vi "Process.vi"(8 "error in":errorcluster, 11 "Instrument.Cryostation UI":refnum<class "Instrument UI.Cryostation.lvclass">) -> (0 "error out":errorcluster, 3 "Instrument.Cryostation UI":refnum<class "Instrument UI.Cryostation.lvclass">)   [LabVIEW 2020, in "Instrument UI.Cryostation.lvclass"]
doc: "---------------------------------------------------------------\nJKI State Machine Objects™\nhttp://jki.net/state-machine-objects/\nCopyright (C) 2005-2015, JKI <info@jki.net>\nALL RIGHTS RESERVEDJKI State Machine Objects (SMO) 1.0.0.5\nJKI - JKI\nCopyright (c) 2016, JKI"
uses:
  Instrument UI.Cryostation.lvclass
  C:/Program Files (x86)/National Instruments/LabVIEW 2020/vi.lib/JKI/JKI SMO/SMO/SMO.lvclass
  C:/Program Files (x86)/National Instruments/LabVIEW 2020/user.lib/LevyLab/Instrument Framework/Instrument UI/Instrument UI.lvclass
  C:/Program Files (x86)/National Instruments/LabVIEW 2020/vi.lib/JKI/JKI SMO/SMO.UI/SMO.UI.lvclass
  instrument.Cryostation/Typedefs/Cryostation.getAll--cluster.ctl
  instrument.Cryostation/instrument.Cryostation.lvclass
  C:/Program Files (x86)/National Instruments/LabVIEW 2020/user.lib/LevyLab/Instrument Framework/Instrument/Instrument.lvclass
  <userlib>/LevyLab/Instrument Framework/Instrument UI/Instrument UI.lvclass/Instrument UI.ctl
  instrument.Cryostation/instrument.Cryostation.lvclass/instrument.Cryostation.ctl
  <vilib>/JKI/JKI SMO/SMO/SMO.lvclass/SMO.ctl
  fdd1bc94-5494-416e-8b24-9b7f0f20f078.vi
  fdd1bc94-5494-416e-8b24-9b7f0f20f078.vi/9c58c222-23e3-43d9-b644-b9682e939e3b.vi
  fdd1bc94-5494-416e-8b24-9b7f0f20f078.vi/ae596761-01aa-4433-afa8-424f3b97f88e.vi
  <vilib>/JKI/JKI SMO/SMO/Private/ReftoDVR--SMO.vi
  <vilib>/Utility/Data Type/Get Type Information.vi
  <vilib>/JDP Science/JSONtext/JSON text to Variant.vi
  <vilib>/JDP Science/JSONtext/LVClass Serializer/JSONtext LVClass Serializer.lvclass
  <userlib>/LevyLab/Instrument Framework/Instrument/Instrument.lvclass
  <userlib>/LevyLab/Instrument Framework/Instrument UI/Instrument UI.lvclass
  Instrument UI.Cryostation.lvclass/Instrument UI.Cryostation.ctl
  <vilib>/JKI/JKI SMO/SMO/SMO.lvclass
  <vilib>/JKI/JKI SMO/SMO.UI/SMO.UI.lvclass
  <userlib>/_OpenG.lib/appcontrol/appcontrol.llb/openg_application_control.lvlib
  D:/Montana-Instruments-Cryostation/lvsrc/instrument.Cryostation UI/Instrument UI.Cryostation.lvclass
  C:/Program Files (x86)/National Instruments/LabVIEW 2020/user.lib/LevyLab/Instrument Framework/Instrument Types/Cryostat/Instrument.Cryostat.lvclass
  D:/Montana-Instruments-Cryostation/lvsrc/instrument.Cryostation/instrument.Cryostation.lvclass
panel:
  out "version":string
  out "Chamber Pressure (mTorr)":dbl=305.0156 format="%#_5f"
  out "Stage 2 Temperature (K)":dbl=305.0156 format="%#_5f"
  out "Stage 1 Temperature (K)":dbl=305.0156 format="%#_5f"
  out "Sample Temperature (K)":dbl=305.0156 format="%#_5f"
  out "Platform Temperature (K)":dbl=305.0156 format="%#_5f"
  # "Cryostation Monitor and Control"
  # "SMO UI Template"
  # "For instructions on how to use the JKI State Machine Objects, examples and video tutorials, visit:\nhttp://jki.net/state-machine-objects/\n\nJKI State Machine Objects™\nhttp://jki.net/state-machine-objects/\nCopyright (C) 2005-2015, JKI <info@jki.net>\nALL RIGHTS RESERVED"
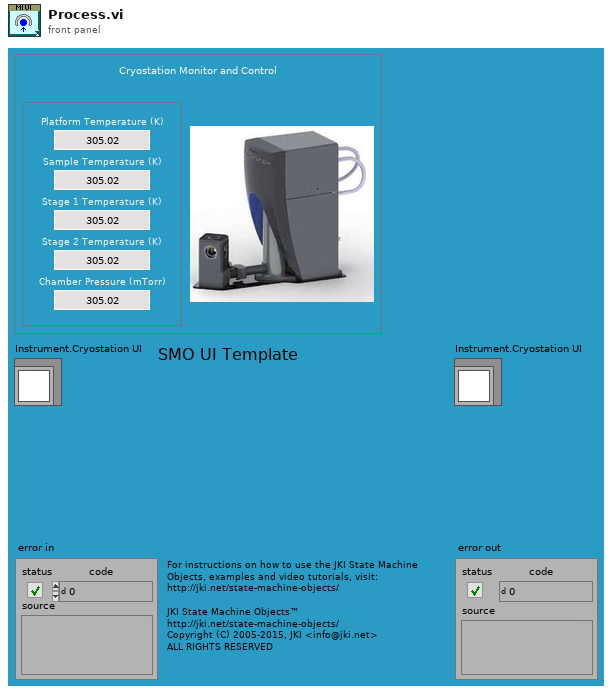
[diagram p1: front panel]
types:
  T1 = enum32{"invalid app kind", "Development System", "Run Time System", "Student Edition", "Embedded LabVIEW", "Evaluation", "Custom"}
  T2 = enum32{"Invalid", "Standard", "Closed", "Hidden", "Minimized", "Maximized"}
  T3 = typedef "instrument.Cryostation.lvclass/Cryostation.getAll--cluster.ctl" = cluster{"Chamber Pressure (mTorr)":dbl, "Compressor Return Pressure (MPa)":dbl, "Compressor Supply Pressure (MPa)":dbl, "Compressor Speed (Hz)":dbl, "Cold Head Speed (Hz)":dbl, "Platform Heater Power (W)":dbl, "Platform Stability (K)":dbl, "Platform Temperature (K)":dbl, "Stage 1 Heater Power (W)":dbl, "Stage 1 Temperature (K)":dbl, "Stage 2 Heater Power (W)":dbl, "Stage 2 Temperature (K)":dbl, "Sample Stability (K)":dbl, "Sample Temperature (K)":dbl, "Temperature Set Point (K)":dbl, "User Stability (K)":dbl, "User Temperature (K)":dbl, "User Temperature Set Point (K)":dbl, "Alarm State":string, "Compressor Run State":string, "Case Valve State":string, "Idle State":string, "Nitrogen State":string, "Vent Valve State":string}
  T4 = cluster{"Core":cluster{"Current VI Reference":refnum<vi>, "Close Panel on Exit?":bool, "Last Error":cluster{"error":errorcluster, "previous state":string, "remaining states":string}, "Shutdown?":bool}, "SelfRef":refnum<class "Instrument UI.Cryostation.lvclass">, "Instrument":refnum<class "instrument.Cryostation.lvclass">, "getAll":T3}
  T5 = cluster{"Current VI Reference":refnum<vi>, "Close Panel on Exit?":bool, "Last Error":cluster{"error":errorcluster, "previous state":string, "remaining states":string}, "Shutdown?":bool}
  T6 = typedef "SMO.lvclass/Protected Events.ctl" = cluster{"StopProcesses":refnum<user-event>, "AbortProcesses":refnum<user-event>, "Config Changed":refnum<user-event>, "Dependency":refnum<user-event>}
  T7 = typedef "Instrument.lvlib/Instrument.lvclass/PublicEvents--Cluster.ctl" = cluster{"MessageFromProcess":refnum<user-event>}
  T8 = typedef "instrument.Cryostation.lvclass/PublicEvents--Cluster.ctl" = cluster{"MessageFromProcess":refnum<user-event>}
  T9 = cluster{"error":errorcluster, "previous state":string, "remaining states":string}
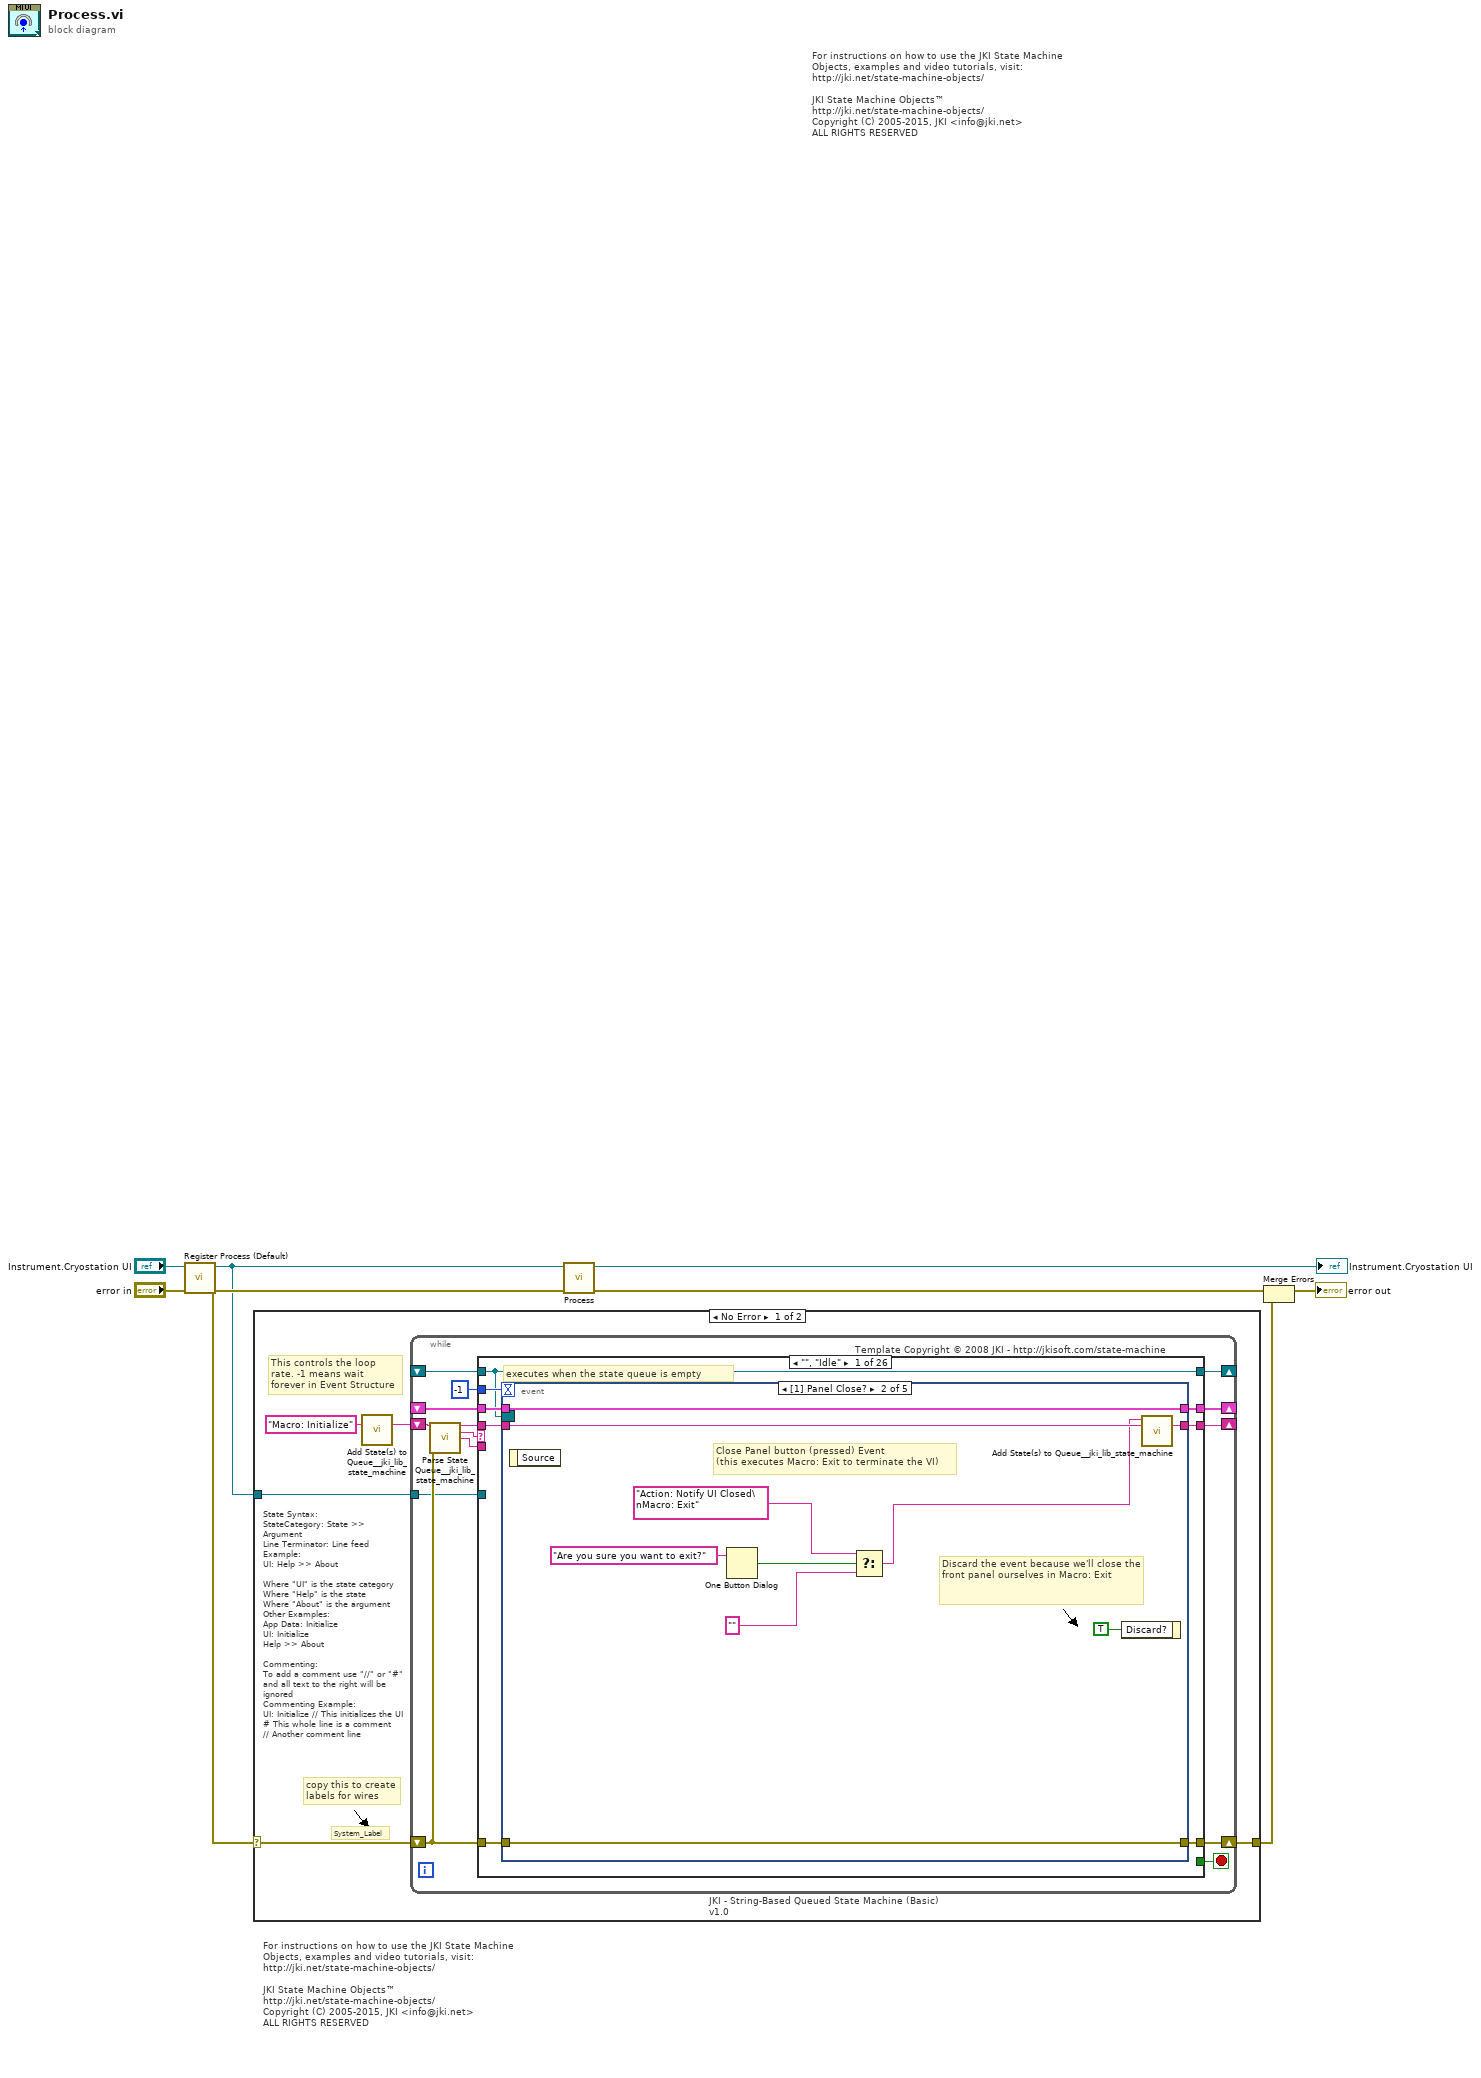
[diagram p0: block diagram]
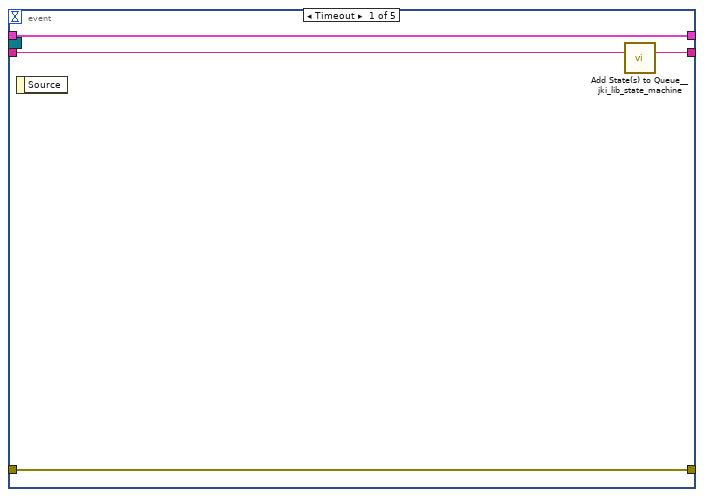
[diagram p2: hidden frame]
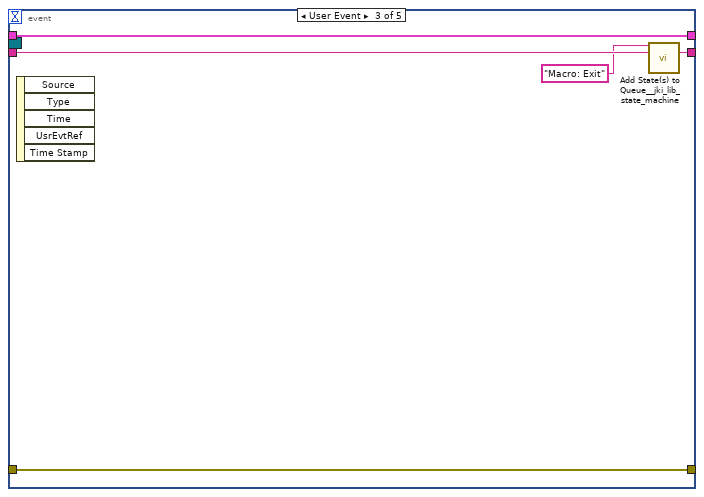
[diagram p3: hidden frame]
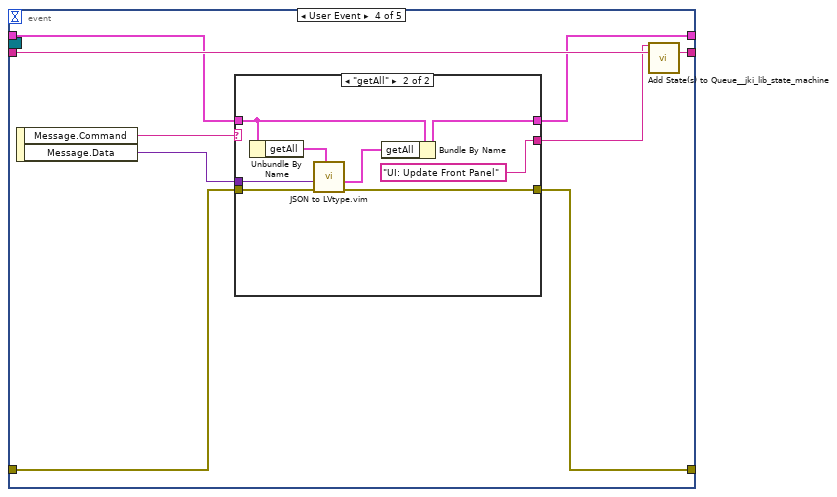
[diagram p4: hidden frame]
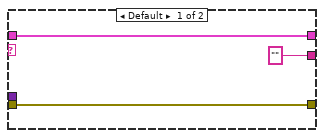
[diagram p5: hidden frame]
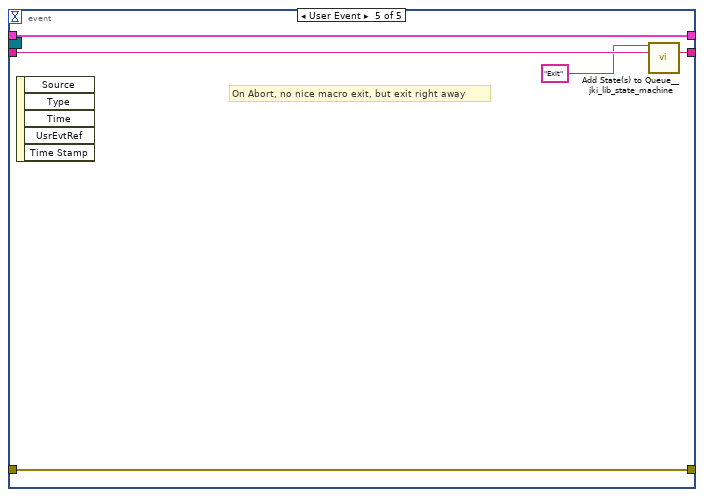
[diagram p6: hidden frame]
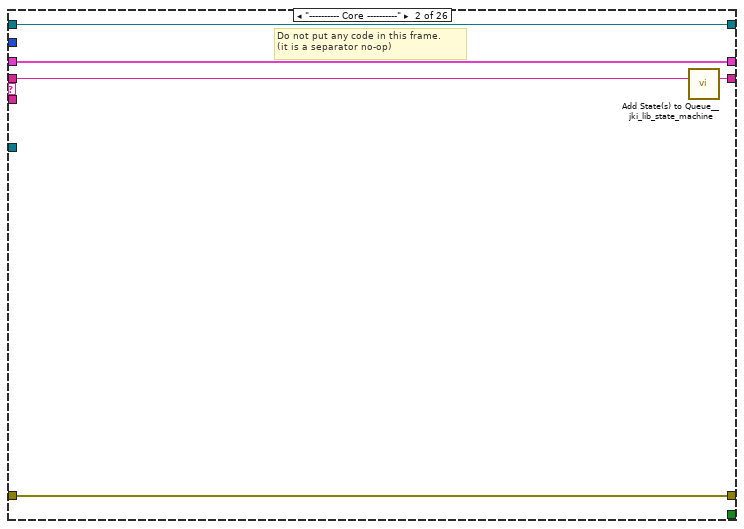
[diagram p7: hidden frame]
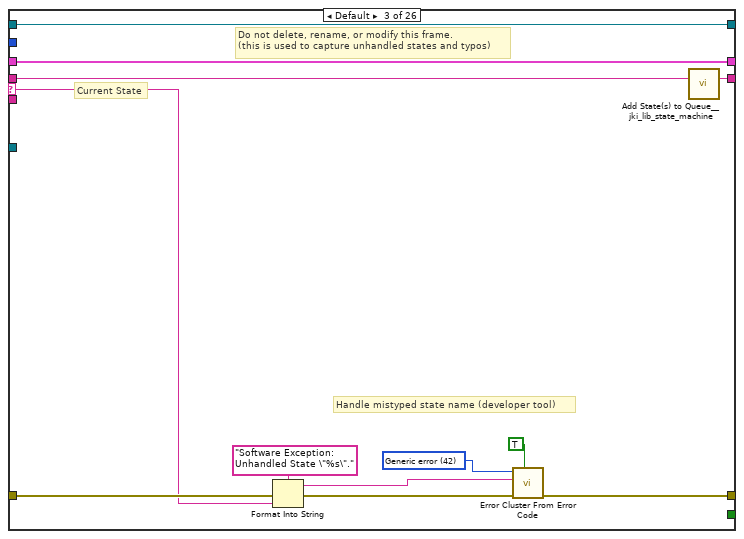
[diagram p8: hidden frame]
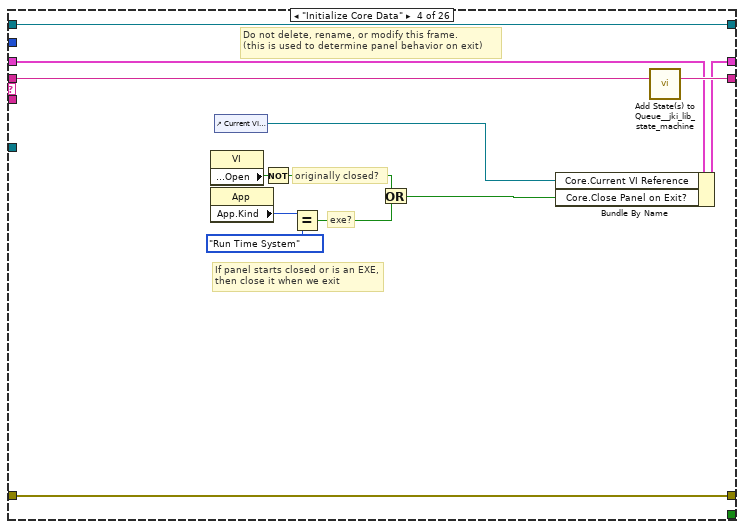
[diagram p9: hidden frame]
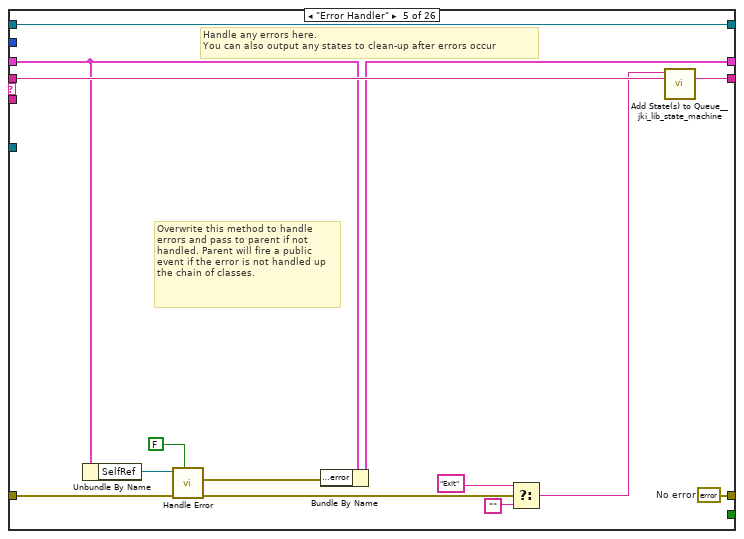
[diagram p10: hidden frame]
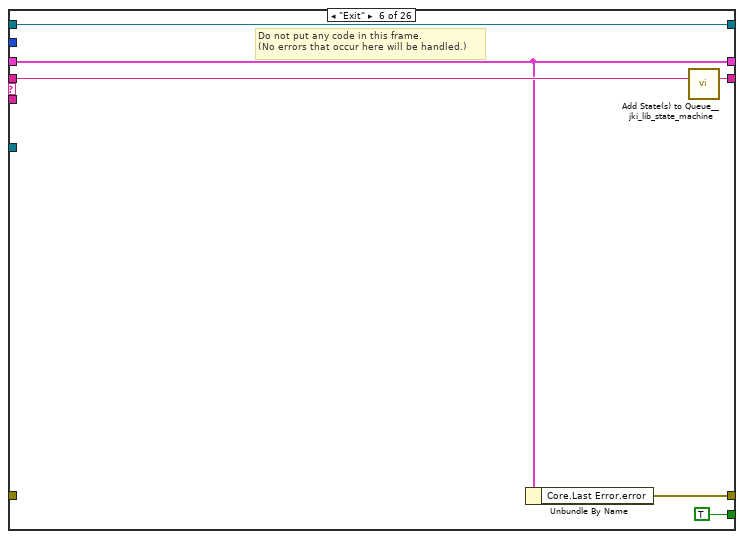
[diagram p11: hidden frame]
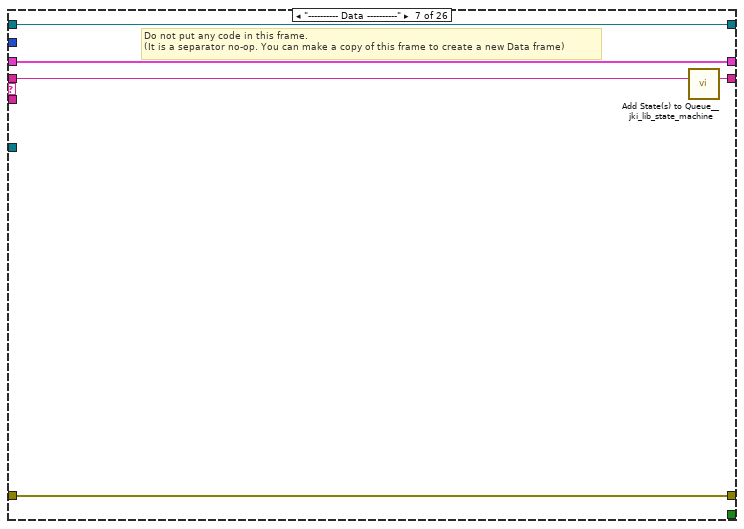
[diagram p12: hidden frame]
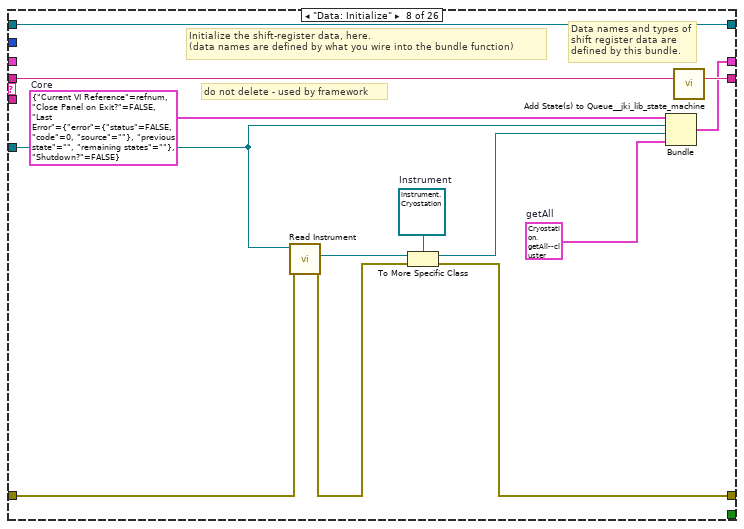
[diagram p13: hidden frame]
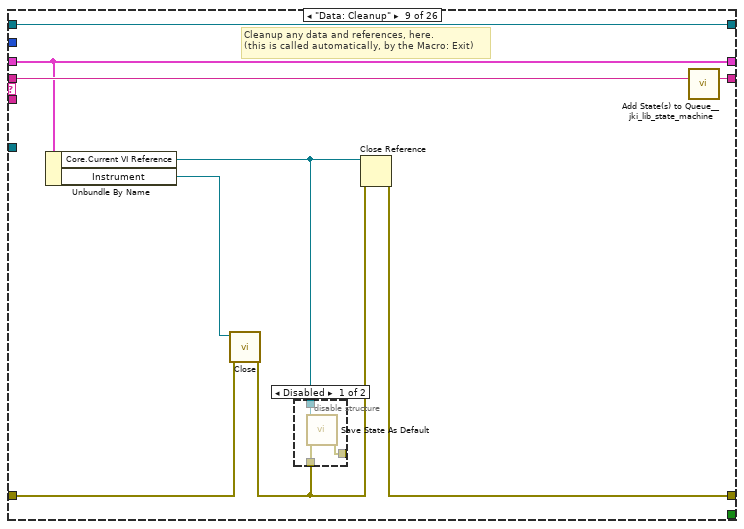
[diagram p14: hidden frame]
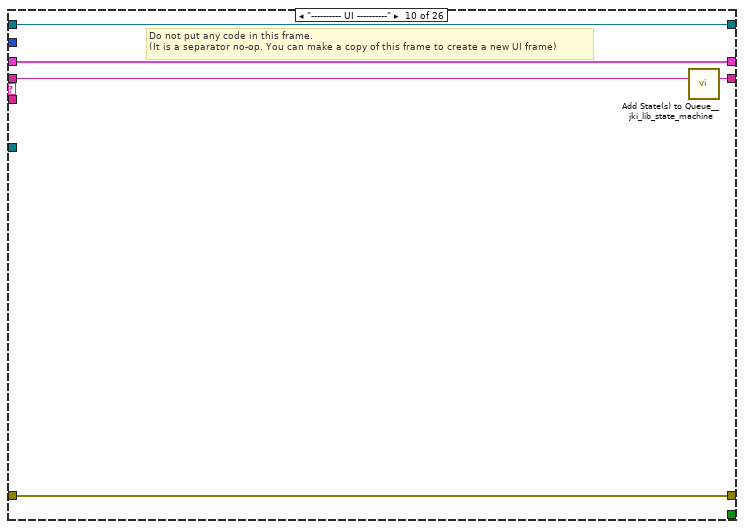
[diagram p16: hidden frame]
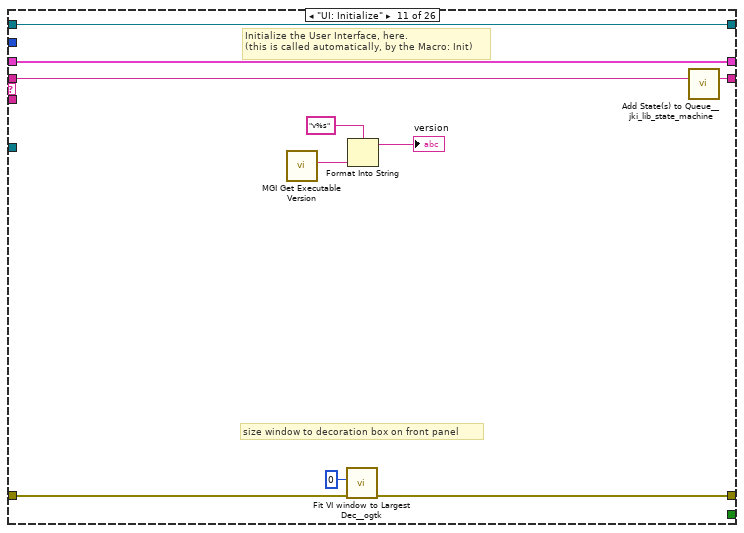
[diagram p17: hidden frame]
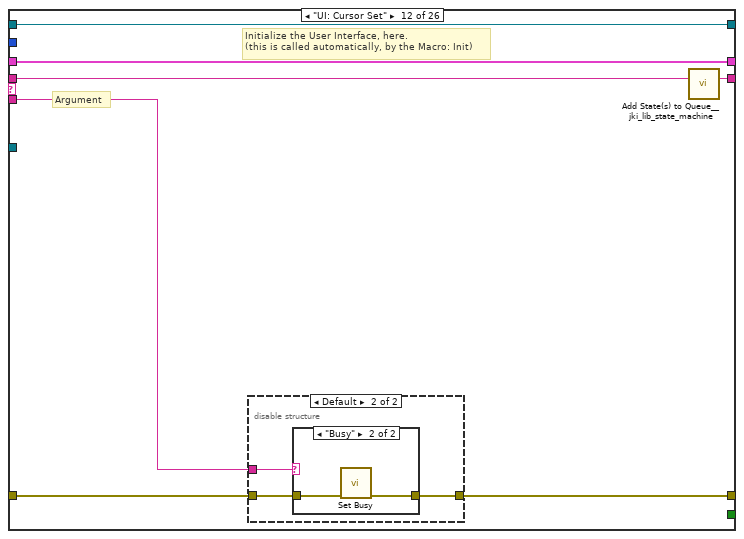
[diagram p18: hidden frame]
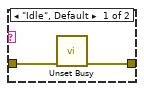
[diagram p20: hidden frame]
diagram:
  # "For instructions on how to use the JKI State Machine Objects, examples and video tutorials, visit:\nhttp://jki.net/state-machine-objects/\n\nJKI State Machine Objects™\nhttp://jki.net/state-machine-objects/\nCopyright (C) 2005-2015, JKI <info@jki.net>\nALL RIGHTS RESERVED"
  # "For instructions on how to use the JKI State Machine Objects, examples and video tutorials, visit:\nhttp://jki.net/state-machine-objects/\n\nJKI State Machine Objects™\nhttp://jki.net/state-machine-objects/\nCopyright (C) 2005-2015, JKI <info@jki.net>\nALL RIGHTS RESERVED"
  n1 = call <vilib>:"Register Process (Default).vi"("error in (no error)"="error in", "SMO"="Instrument.Cryostation UI") -> ("error out"=w5:errorcluster, "SelfRef"=w4:refnum<class "Instrument UI.Cryostation.lvclass">)  [unwired: 8 in]
  n2 = case shown="No Error" w5 {
    selector: w5 -> [w10 w335]
    tunnel: w4 -> [w11 _]
    tunnel: [w9 w335] -> w1
    frame No Error {
      # "State Syntax:\nStateCategory: State >> Argument\nLine Terminator: Line feed\nExample:\nUI: Help >> About\n\nWhere \"UI\" is the state category\nWhere \"Help\" is the state\nWhere \"About\" is the argument\nOther Examples:\nApp Data: Initialize\nUI: Initialize\nHelp >> About\n\nCommenting:\nTo add a comment use \"//\" or \"#\" and all text to the right will be ignored\nCommenting Example:\nUI: Initialize // This initializes the UI\n# This whole line is a comment\n// Another comment line"
      # "copy this to create labels for wires"
      # "This controls the loop rate. -1 means wait forever in Event Structure"
      # "System_Label"
      n3 = call <vilib>:"Add State(s) to Queue__jki_lib_state_machine.vi"("State(s) in (\"\")"="Macro: Initialize") -> ("States Out"=w13:string)  [unwired: 14 in]
      n4 = while "JKI - String-Based Queued State Machine (Basic) v1.0" {
        shift-right: [w20] -> _
        shift-left: _ -> [w19]
        shift-right: [w23] -> w9
        shift-left: w10 -> [w17]
        shift-right: [w22] -> _
        shift-left: w13 -> [w24]
        tunnel: w11 -> [w16]
        shift-right: [w15] -> _
        shift-left: _ -> [w14]
        stop <- w21 stop-if-true
        # "Template Copyright © 2008 JKI - http://jkisoft.com/state-machine"
        n5 = call <vilib>:"Parse State Queue__jki_lib_state_machine.vi"("State Queue"=w24, "Error In (no error)"=w17) -> ("Remaining States"=w26:string, "Current State"=w27:string, "Arguments"=w25:string)  [unwired: 11 in]
        n6 = case shown="\"\", \"Idle\"" w27 {
          selector: w27 -> [_ _ w86 _ _ _ _ _ _ _ _ _ _ _ _ _ _ _ _ _ _ _ _ _ _ _]
          tunnel: w26 -> [w35 w84 w90 w109 w123 w129 w134 w147 w156 w164 w174 w181 w197 w235 w240 w249 w263 w268 w279 w286 w293 w298 w314 w320 w327 w334]
          tunnel: w25 -> [_ _ _ _ _ _ _ _ _ _ _ w175 w191 _ _ _ _ _ _ _ _ _ _ _ _ _]
          tunnel: w19 -> [w33 w81 w88 w100 w111 w125 w131 _ w151 w161 w172 w179 w193 w232 w237 w245 w254 w265 w276 w281 w290 w295 w312 w318 w323 w330]
          tunnel: [w32 w82 w92 w106 w116 w124 w132 w139 w154 w162 w169 w176 w194 w231 w238 w247 w261 w266 w270 w282 w287 w296 w309 w315 w324 w328] -> w23
          tunnel: w17 -> [w31 w82 w91 w106 w112 _ w132 w136 w149 w162 w170 w177 w195 w231 w238 w247 w261 w266 w271 w283 w288 w296 w299 w316 w324 w329]
          tunnel: [w34 w83 w89 w108 w122 w128 w133 w146 w155 w163 w173 w180 w196 w234 w239 w248 w262 w267 w278 w285 w292 w297 w313 w319 w326 w333] -> w22
          tunnel: [_ _ _ _ _ TRUE _ _ _ _ _ _ _ _ _ _ _ _ _ _ _ _ _ _ _ _] -> w21
          tunnel: [w30 w81 w88 w107 w114 w125 w131 w145 w151 w161 w172 w179 w193 w232 w237 w245 w254 w265 w276 w281 w290 w295 w312 w318 w322 w330] -> w20
          tunnel: -1 ("Timeout") -> [w29 _ _ _ _ _ _ _ _ _ _ _ _ _ _ _ _ _ _ _ _ _ _ _ _ _]
          tunnel: w16 -> [_ _ _ _ _ _ _ w135 _ _ _ _ _ _ _ _ _ _ _ _ _ _ _ _ _ _]
          tunnel: [w28 w80 w85 w97 w121 w126 w130 w144 w153 w160 w171 w178 w190 w233 w236 w246 w255 w264 w277 w284 w291 w294 w311 w317 w325 w332] -> w15
          tunnel: w14 -> [w28 w80 w85 w97 w121 w126 w130 w144 w153 w160 w171 w178 w190 w233 w236 w246 w255 w264 w277 w284 w291 w294 _ w317 w325 w332]
          frame "", "Idle" {
            # "executes when the state queue is empty"
            n7 = event shown="[1] Panel Close?" {
              selector: w28 -> [_ _ _ _ _]
              dyn-events: _ -> [_ _ _ _ _]
              timeout: w29 -> [_ _ _ _ _]
              tunnel: w35 -> [w39 w49 w54 w63 w79]
              tunnel: [w38 w48 w53 w62 w78] -> w34
              tunnel: w33 -> [w36 w46 w51 w58 w76]
              tunnel: [w37 w45 w52 w57 w77] -> w32
              tunnel: w31 -> [w37 w45 w52 w59 w77]
              tunnel: [w36 w46 w51 w60 w76] -> w30
              event Timeout {
                n8 = event-data() -> ()  [unwired: 1 in, 1 out]
                n9 = call <vilib>:"Add State(s) to Queue__jki_lib_state_machine.vi"("State(s) in (\"\")"=w39) -> ("States Out"=w38:string)  [unwired: 14 in]
              }
              event Panel Close? {
                # "Discard the event because we'll close the front panel ourselves in Macro: Exit"
                # "Close Panel button (pressed) Event\n(this executes Macro: Exit to terminate the VI)"
                n10 = event-data() -> ()  [unwired: 1 in, 1 out]
                n11 = One Button Dialog(message="Are you sure you want to exit?") -> (true=w44:bool)  [unwired: 1 in]
                n12 = Select(t="Action: Notify UI Closed\nMacro: Exit", s=w44, f="") -> (s? t:f=w41:string)
                n13 = event-data("Discard?"=TRUE) -> ()  [unwired: 1 in, 1 out]
                n14 = call <vilib>:"Add State(s) to Queue__jki_lib_state_machine.vi"("State(s) in Front (\"\")"=w41, "State(s) in (\"\")"=w49) -> ("States Out"=w48:string)  [unwired: 13 in]
              }
              event User Event {
                n15 = event-data() -> ()  [unwired: 1 in, 5 out]
                n16 = call <vilib>:"Add State(s) to Queue__jki_lib_state_machine.vi"("State(s) in Front (\"\")"="Macro: Exit", "State(s) in (\"\")"=w54) -> ("States Out"=w53:string)  [unwired: 13 in]
              }
              event User Event {
                n17 = event-data() -> ("Message.Command"=w56:string, "Message.Data"=w61:variant)  [unwired: 1 in]
                n18 = case shown="\"getAll\"" w56 {
                  tunnel: w61 -> [_ w74]
                  tunnel: [w66 w71] -> w60
                  tunnel: w59 -> [w64 w70]
                  tunnel: w58 -> [w66 w69]
                  tunnel: [w64 w68] -> w57
                  tunnel: ["" "UI: Update Front Panel"] -> w55
                  frame Default {
                  }
                  frame "getAll" {
                    n19 = Unbundle By Name(w69) -> ("getAll"=w73:T3)
                    n20 = call "JSON to LVtype.vim"("type"=w73, "error in (no error)"=w70, "JSON Data in"=w74) -> ("error out"=w68:errorcluster, "Data out"=w72:T3)  [unwired: 7 in]
                    n21 = Bundle By Name(cluster=w69, "getAll"=w72) -> (w71:T4)
                  }
                }
                n22 = call <vilib>:"Add State(s) to Queue__jki_lib_state_machine.vi"("State(s) in Front (\"\")"=w55, "State(s) in (\"\")"=w63) -> ("States Out"=w62:string)  [unwired: 13 in]
              }
              event User Event {
                # "On Abort, no nice macro exit, but exit right away"
                n23 = event-data() -> ()  [unwired: 1 in, 5 out]
                n24 = call <vilib>:"Add State(s) to Queue__jki_lib_state_machine.vi"("State(s) in Front (\"\")"="Exit", "State(s) in (\"\")"=w79) -> ("States Out"=w78:string)  [unwired: 13 in]
              }
            }
          }
          frame "---------- Core ----------" {
            # "Do not put any code in this frame.\n(it is a separator no-op)"
            n25 = call <vilib>:"Add State(s) to Queue__jki_lib_state_machine.vi"("State(s) in (\"\")"=w84) -> ("States Out"=w83:string)  [unwired: 14 in]
          }
          frame Default {
            w95 = 42 items=["No error", "Argument error", "Memory is full", "Out of zone", "End of file", "File already open", "Generic file I/O error", "File not found", "File permission error", "Disk is full", "Duplicate path", "Too many files open", "System feature not enabled", "Resource file not found", "Cannot add resource", "Resource not found", "Image not found", "Image memory error", "Pen does not exist", "Config type invalid", "Config token not found", "Config parse error", "Config memory error", "Bad external code format", "Bad external code offset", "External code not present", "Null window", "Destroy window error", "Null menu", "Print aborted", "Bad print record", "Print driver error", "Windows error during printing", "Memory error during printing", "Print dialog error", "Generic print error", "Invalid device refnum", "Device not found", "Device parameter error", "Device unit error", "Cannot open device", "Device call aborted", "Generic error", "Cancelled by user", "Object ID too low", "Object ID too high", "Object not in heap", "Unknown heap", "Unknown object (invalid DefProc)", "Unknown object (DefProc not in table)", "Message out of range", "Invalid (null) method", "Unknown message", "Manager call not supported", "Bad address", "Network operation in progress", "Network operation timed out", "Connection is busy", "Network attribute not supported", "Network error", "Address in use", "System out of memory", "Connection aborted", "Connection refused", "Not connected", "Already connected", "Connection closed", "Initialization error (interapplication manager)", "Bad occurrence", "Wait on unbound occurrence handler", "Occurrence queue overflow", "Datalog type conflict", "Unused", "Unrecognized type (interapplication manager)", "Memory corrupt", "Failed to make temporary DLL", "Old CIN version", "Drag socket not found", "Failed to load drop-object", "Failed to register OLE object", "Failed to release OLE object", "Format specifier type mismatch", "Unknown format specifier", "Too few format specifiers", "Too many format specifiers", "Scan failed", "Newer CIN version", "Error converting to variant", "Runtime menu error", "Password tampered", "Variant attribute not found", "Incompatible variant data type", "Event data is not available", "Event Store is not present", "Occurrence is not found", "Event Queue is not created", "Event info is not available", "Refnum passed is NULL", "Error retrieving Class GUID", "Error retrieving CoClass GUID", "Error retrieving TypeLib GUID.", "Bad built application magic bytes.", "Specific driver is different from the specific driver associated with the Logical Name.", "There is no session opened to the class driver.", "Max Error", "MAX - Error with config objects", "MAX - Error loading configuration", "MAX - Group not supported"]
            # "Current State"
            # "Do not delete, rename, or modify this frame.\n(this is used to capture unhandled states and typos)"
            # "Handle mistyped state name (developer tool)"
            n26 = Format Into String(format string="Software Exception: Unhandled State \"%s\"." ("message"), error in=w91, w86) -> (resulting string=w94:string, error out=w93:errorcluster)  [unwired: 1 in]
            n27 = call <vilib>:"Error Cluster From Error Code.vi"("show call chain? (False)"=TRUE, "error in (no error)"=w93, "error message (\"\")"=w94, "error code (0)"=w95) -> ("error out"=w92:errorcluster)  [unwired: 5 in]
            n28 = call <vilib>:"Add State(s) to Queue__jki_lib_state_machine.vi"("State(s) in (\"\")"=w90) -> ("States Out"=w89:string)  [unwired: 14 in]
          }
          frame "Initialize Core Data" {
            # "Do not delete, rename, or modify this frame.\n(this is used to determine panel behavior on exit)"
            # "originally closed?"
            # "exe?"
            # "If panel starts closed or is an EXE, then close it when we exit"
            n29 = property class="VI"() -> ("Front Panel.Open"=w105:bool)  [unwired: 2 in, 2 out]
            n30 = property class="App"() -> ("App.Kind"=w104:T1)  [unwired: 2 in, 2 out]
            n31 = control-ref of="Current VI Reference"() -> (w98:refnum<vi>)
            n32 = Not(x=w105) -> (.not. x?=w102:bool)
            n33 = Equal?(x=w104, y=T1."Run Time System" ("Application:Kind")) -> (x = y?=w101:bool)
            n34 = Or(x=w102, y=w101) -> (x .or. y?=w99:bool)
            n35 = Bundle By Name(cluster=w100, "Core.Current VI Reference"=w98, "Core.Close Panel on Exit?"=w99) -> (w107:T4)
            n36 = call <vilib>:"Add State(s) to Queue__jki_lib_state_machine.vi"("State(s) in (\"\")"=w109) -> ("States Out"=w108:string)  [unwired: 14 in]
          }
          frame "Error Handler" {
            w116 = errorcluster {"status"=FALSE, "code"=0, "source"=""}  # No error
            # "Overwrite this method to handle errors and pass to parent if not handled. Parent will fire a public event if the error is not handled up the chain of classes."
            # "Handle any errors here.\nYou can also output any states to clean-up after errors occur"
            n37 = Unbundle By Name(w111) -> ("SelfRef"=w120:refnum<class "Instrument UI.Cryostation.lvclass">)
            n38 = call-dynamic "Handle Error.vi"("Stop on Unhandled Error (T)"=FALSE, "error in"=w112, "SMO"=w120) -> ("handling error"=w110:errorcluster, "Unhandled error"=w115:errorcluster)  [unwired: 6 in, 1 out]
            n39 = Bundle By Name(cluster=w111, "Core.Last Error.error"=w115) -> (w114:T4)
            n40 = Select(t="Exit", s=w110, f="") -> (s? t:f=w117:string)
            n41 = call <vilib>:"Add State(s) to Queue__jki_lib_state_machine.vi"("State(s) in Front (\"\")"=w117, "State(s) in (\"\")"=w123) -> ("States Out"=w122:string)  [unwired: 13 in]
          }
          frame "Exit" {
            # "Do not put any code in this frame.\n(No errors that occur here will be handled.)"
            n42 = Unbundle By Name(w125) -> ("Core.Last Error.error"=w124:errorcluster)
            n43 = call <vilib>:"Add State(s) to Queue__jki_lib_state_machine.vi"("State(s) in (\"\")"=w129) -> ("States Out"=w128:string)  [unwired: 14 in]
          }
          frame "---------- Data ----------" {
            # "Do not put any code in this frame.\n(It is a separator no-op. You can make a copy of this frame to create a new Data frame)"
            n44 = call <vilib>:"Add State(s) to Queue__jki_lib_state_machine.vi"("State(s) in (\"\")"=w134) -> ("States Out"=w133:string)  [unwired: 14 in]
          }
          frame "Data: Initialize" {
            w141 = refnum<class "instrument.Cryostation.lvclass"> refnum  # Instrument
            w142 = T3 {"Chamber Pressure (mTorr)"=0.0, "Compressor Return Pressure (MPa)"=0.0, "Compressor Supply Pressure (MPa)"=0.0, "Compressor Speed (Hz)"=0.0, "Cold Head Speed (Hz)"=0.0, "Platform Heater Power (W)"=0.0, "Platform Stability (K)"=0.0, "Platform Temperature (K)"=0.0, "Stage 1 Heater Power (W)"=0.0, "Stage 1 Temperature (K)"=0.0, "Stage 2 Heater Power (W)"=0.0, "Stage 2 Temperature (K)"=0.0, "Sample Stability (K)"=0.0, "Sample Temperature (K)"=0.0, "Temperature Set Point (K)"=0.0, "User Stability (K)"=0.0, "User Temperature (K)"=0.0, "User Temperature Set Point (K)"=0.0, "Alarm State"="", "Compressor Run State"="", "Case Valve State"="", "Idle State"="", "Nitrogen State"="", "Vent Valve State"=""}  # getAll
            w143 = T5 {"Current VI Reference"=refnum, "Close Panel on Exit?"=FALSE, "Last Error"={"error"={"status"=FALSE, "code"=0, "source"=""}, "previous state"="", "remaining states"=""}, "Shutdown?"=FALSE}  # Core
            # "do not delete - used by framework"
            # "Data names and types of shift register data are defined by this bundle."
            # "Initialize the shift-register data, here.\n(data names are defined by what you wire into the bundle function)"
            n45 = call <userlib>:"Read Instrument.vi"("error in (no error)"=w136, "Instrument UI in"=w135) -> ("error out"=w137:errorcluster, "Instrument"=w138:refnum<class "Instrument.lvclass">)  [unwired: 7 in, 1 out]
            n46 = To More Specific Class(target class=w141, reference=w138, error in=w137) -> (specific class reference=w140:refnum<class "instrument.Cryostation.lvclass">, error out=w139:errorcluster)
            n47 = Bundle("Core"=w143, "SelfRef"=w135, "Instrument"=w140, "getAll"=w142) -> (w145:T4)  [unwired: 1 in]
            n48 = call <vilib>:"Add State(s) to Queue__jki_lib_state_machine.vi"("State(s) in (\"\")"=w147) -> ("States Out"=w146:string)  [unwired: 14 in]
          }
          frame "Data: Cleanup" {
            # "Cleanup any data and references, here.\n(this is called automatically, by the Macro: Exit)"
            n49 = Unbundle By Name(w151) -> ("Core.Current VI Reference"=w152:refnum<vi>, "Instrument"=w150:refnum<class "instrument.Cryostation.lvclass">)
            n50 = call-dynamic "Close.vi"("error in (no error)"=w149, "instrument.Cryostation in"=w150) -> ("error out"=w148:errorcluster)  [unwired: 8 in, 1 out]
            n51 = disable-structure shown="Disabled" {
              disable-tunnel: w152 -> [w159 _]
              disable-tunnel: [w158 _] -> _
              disable-tunnel: w148 -> [w157 _]
              frame Disabled {
                n52 = call <vilib>:"Save State As Default.vi"("Error In"=w157, "Target VI"=w159) -> ("Error Out"=w158:errorcluster)  [unwired: 8 in, 1 out]
              }
              frame Enabled {
              }
            }
            n53 = Close Reference(reference=w152, error in (no error)=w148) -> (error out=w154:errorcluster)
            n54 = call <vilib>:"Add State(s) to Queue__jki_lib_state_machine.vi"("State(s) in (\"\")"=w156) -> ("States Out"=w155:string)  [unwired: 14 in]
          }
          frame "---------- UI ----------" {
            # "Do not put any code in this frame.\n(It is a separator no-op. You can make a copy of this frame to create a new UI frame)"
            n55 = call <vilib>:"Add State(s) to Queue__jki_lib_state_machine.vi"("State(s) in (\"\")"=w164) -> ("States Out"=w163:string)  [unwired: 14 in]
          }
          frame "UI: Initialize" {
            # "size window to decoration box on front panel"
            # "Initialize the User Interface, here.\n(this is called automatically, by the Macro: Init)"
            n56 = call <userlib>:"MGI Get Executable Version.vi"() -> ("Version"=w167:string)  [unwired: 7 in]
            n57 = call <userlib>:"Fit VI window to Largest Dec__ogtk.vi"("error in (no error)"=w170, "border spacing (2 px)"=0) -> ("error out"=w169:errorcluster)  [unwired: 4 in, 1 out]
            n58 = Format Into String(format string="v%s", w167) -> (resulting string=→"version":string)  [unwired: 2 in, 1 out]
            n59 = call <vilib>:"Add State(s) to Queue__jki_lib_state_machine.vi"("State(s) in (\"\")"=w174) -> ("States Out"=w173:string)  [unwired: 14 in]
          }
          frame "UI: Cursor Set" {
            # "Argument"
            # "Initialize the User Interface, here.\n(this is called automatically, by the Macro: Init)"
            n60 = disable-structure shown="Default" {
              disable-tunnel: w177 -> [w182 w185]
              disable-tunnel: [w182 w184] -> w176
              disable-tunnel: w175 -> [_ w183]
              frame condition #0 {
              }
              frame condition #1 (active) {
                n61 = case shown="\"Busy\"" w183 {
                  tunnel: w185 -> [w187 w189]
                  tunnel: [w186 w188] -> w184
                  frame "Idle", Default {
                    n62 = call <vilib>:"Unset Busy.vi"("error in (no error)"=w187) -> ("error out"=w186:errorcluster)  [unwired: 10 in]
                  }
                  frame "Busy" {
                    n63 = call <vilib>:"Set Busy.vi"("error in (no error)"=w189) -> ("error out"=w188:errorcluster)  [unwired: 9 in, 1 out]
                  }
                }
              }
            }
            n64 = call <vilib>:"Add State(s) to Queue__jki_lib_state_machine.vi"("State(s) in (\"\")"=w181) -> ("States Out"=w180:string)  [unwired: 14 in]
          }
          frame "UI: Front Panel State" {
            # "Argument"
            # "Set Front Panel Open or Closed\n(Usage: \"UI: Front Panel State >> Open|Close\")"
            n65 = Unbundle By Name(w193) -> ("Core.Current VI Reference"=w192:refnum<vi>)
            n66 = disable-structure shown="Default" {
              disable-tunnel: w195 -> [w201 w224]
              disable-tunnel: [w200 w224] -> w194
              disable-tunnel: w192 -> [w199 _]
              disable-tunnel: w191 -> [w198 _]
              frame condition #0 (active) {
                n67 = case shown="\"Close\"" w198 {
                  tunnel: w201 -> [w205 w218]
                  tunnel: [w207 w219] -> w200
                  tunnel: w199 -> [w206 w216]
                  frame "Open", Default {
                    n68 = property class="VI"(reference=w206, error in=w205) -> (reference out=w203:refnum<vi>, error out=w204:errorcluster, "FP.State"=w202:T2)
                    n69 = case shown="\"Closed\"" w202 {
                      tunnel: [w210 w213] -> w207
                      tunnel: w204 -> [w209 w213]
                      tunnel: w203 -> [w208 _]
                      frame "Closed" {
                        n70 = invoke class="VI" method="FP.Open"(reference=w208, error in=w209, "Activate"=TRUE, "State"=T2."Standard") -> (error out=w210:errorcluster)  [unwired: 1 in, 4 out]
                      }
                      frame Default {
                      }
                    }
                  }
                  frame "Close" {
                    n71 = property class="VI"(reference=w216, error in=w218) -> (reference out=w215:refnum<vi>, error out=w217:errorcluster, "FP.State"=w214:T2)
                    n72 = case shown="Default" w214 {
                      tunnel: [w220 w223] -> w219
                      tunnel: w217 -> [w220 w222]
                      tunnel: w215 -> [_ w221]
                      frame "Invalid", "Closed" {
                      }
                      frame Default {
                        n73 = invoke class="VI" method="FP.Close"(reference=w221, error in=w222) -> (error out=w223:errorcluster)  [unwired: 1 in, 2 out]
                      }
                    }
                  }
                }
              }
              frame condition #1 {
              }
            }
            n74 = call <vilib>:"Add State(s) to Queue__jki_lib_state_machine.vi"("State(s) in (\"\")"=w197) -> ("States Out"=w196:string)  [unwired: 14 in]
          }
          frame "UI: Update Front Panel" {
            n75 = Unbundle By Name(w232) -> ("getAll"=w225:T3)
            n76 = Unbundle By Name(w225) -> ("Platform Temperature (K)"=→"Platform Temperature (K)":dbl, "Sample Temperature (K)"=→"Sample Temperature (K)":dbl, "Stage 1 Temperature (K)"=→"Stage 1 Temperature (K)":dbl, "Stage 2 Temperature (K)"=→"Stage 2 Temperature (K)":dbl, "Chamber Pressure (mTorr)"=→"Chamber Pressure (mTorr)":dbl)
            n77 = call <vilib>:"Add State(s) to Queue__jki_lib_state_machine.vi"("State(s) in (\"\")"=w235) -> ("States Out"=w234:string)  [unwired: 14 in]
          }
          frame "---------- Macro ----------" {
            # "Do not put any code in this frame.\n(It is a separator no-op. You can make a copy of this frame to create a new Macro frame)"
            n78 = call <vilib>:"Add State(s) to Queue__jki_lib_state_machine.vi"("State(s) in (\"\")"=w240) -> ("States Out"=w239:string)  [unwired: 14 in]
          }
          frame "Macro: Initialize" {
            # "Initialization Macro\n(This is called once, when the VI starts)"
            n79 = call <vilib>:"Add State(s) to Queue__jki_lib_state_machine.vi"("State(s) in Front (\"\")"="Data: Initialize\nInitialize Core Data\nEvents: Register", "State(s) in (\"\")"="Process: Sync", "State(s) at Back (\"\")"="UI: Initialize\nUI: Front Panel State >> Open") -> ("States Out"=w242:string)  [unwired: 12 in]
            n80 = call <vilib>:"Add State(s) to Queue__jki_lib_state_machine.vi"("State(s) in Front (\"\")"=w242, "State(s) in (\"\")"=w249) -> ("States Out"=w248:string)  [unwired: 13 in]
          }
          frame "Macro: Exit" {
            # "Exit Macro\n(This is called once, when the VI exits)"
            n81 = Unbundle By Name(w254) -> ("Core.Close Panel on Exit?"=w260:bool)
            n82 = Select(t="UI: Front Panel State >> Close", s=w260, f="") -> (s? t:f=w257:string)
            n83 = call <vilib>:"Add State(s) to Queue__jki_lib_state_machine.vi"("State(s) in Front (\"\")"="Data: Cleanup\nEvents: Unregister\nProcess: Self Terminate", "State(s) in (\"\")"="Process: Sync", "State(s) at Back (\"\")"="Exit") -> ("States Out"=w251:string)  [unwired: 12 in]
            n84 = call <vilib>:"Add State(s) to Queue__jki_lib_state_machine.vi"("State(s) in (\"\")"=w257, "State(s) at Back (\"\")"=w251) -> ("States Out"=w256:string)  [unwired: 13 in]
            n85 = call <vilib>:"Add State(s) to Queue__jki_lib_state_machine.vi"("State(s) in Front (\"\")"=w256, "State(s) in (\"\")"=w263) -> ("States Out"=w262:string)  [unwired: 13 in]
          }
          frame "---------- Process ----------" {
            # "Template Separator\n(You can make a copy of, or modify, this frame)"
            n86 = call <vilib>:"Add State(s) to Queue__jki_lib_state_machine.vi"("State(s) in (\"\")"=w268) -> ("States Out"=w267:string)  [unwired: 14 in]
          }
          frame "Process: Sync" {
            n87 = Unbundle By Name(w276) -> ("SelfRef"=w272:refnum<class "Instrument UI.Cryostation.lvclass">)
            n88 = call <vilib>:"WaitOnProcessSync.vi"("error in (no error)"=w271, "SMO"=w272) -> ("error out"=w270:errorcluster, "Don't run?"=w275:bool)  [unwired: 7 in, 1 out]
            n89 = Select(t="Data: Cleanup\nEvents: Unregister\nExit", s=w275, f="") -> (s? t:f=w269:string)
            n90 = call <vilib>:"Add State(s) to Queue__jki_lib_state_machine.vi"("State(s) in Front (\"\")"=w269, "State(s) in (\"\")"=w279) -> ("States Out"=w278:string)  [unwired: 13 in]
          }
          frame "Process: Self Terminate" {
            n91 = Unbundle By Name(w281) -> ("SelfRef"=w280:refnum<class "Instrument UI.Cryostation.lvclass">)
            n92 = call <vilib>:"SelfTerminate.vi"("error in (no error)"=w283, "SMO in"=w280) -> ("error out"=w282:errorcluster)  [unwired: 8 in, 1 out]
            n93 = call <vilib>:"Add State(s) to Queue__jki_lib_state_machine.vi"("State(s) in (\"\")"=w286) -> ("States Out"=w285:string)  [unwired: 14 in]
          }
          frame "Process: Stop Instrument" {
            # "Template Separator\n(You can make a copy of, or modify, this frame)"
            n94 = Unbundle By Name(w290) -> ("Instrument"=w289:refnum<class "instrument.Cryostation.lvclass">)
            n95 = call <vilib>:"Stop.vi"("error in (no error)"=w288, "SMO"=w289) -> ("error out"=w287:errorcluster)  [unwired: 8 in, 1 out]
            n96 = call <vilib>:"Add State(s) to Queue__jki_lib_state_machine.vi"("State(s) in (\"\")"=w293) -> ("States Out"=w292:string)  [unwired: 14 in]
          }
          frame "---------- Events ----------" {
            # "Template Separator\n(You can make a copy of, or modify, this frame)"
            n97 = call <vilib>:"Add State(s) to Queue__jki_lib_state_machine.vi"("State(s) in (\"\")"=w298) -> ("States Out"=w297:string)  [unwired: 14 in]
          }
          frame "Events: Register" {
            # "Expand to add\nmore events"
            # "Base Class Protected Events"
            n98 = Unbundle By Name(w312) -> ("SelfRef"=w308:refnum<class "Instrument UI.Cryostation.lvclass">, "Instrument"=w307:refnum<class "instrument.Cryostation.lvclass">)
            n99 = call <vilib>:"GetProtectedEvents.vi"("SMO"=w308) -> ("error out"=w300:errorcluster, "SMO Protected Events"=w310:T6)  [unwired: 8 in, 1 out]
            n100 = call <userlib>:"Instrument.GetPublicEvents.vi"("Instrument"=w307) -> ("error out"=w301:errorcluster, "Instrument Public Events"=w306:T7, "Instrument out"=w304:refnum<class "instrument.Cryostation.lvclass">)  [unwired: 8 in]
            n101 = call "Cryostation.GetPublicEvents.vi"("instrument.Cryostation in"=w304) -> ("error out"=w302:errorcluster, "Cryostation.Public Events"=w305:T8)  [unwired: 8 in, 1 out]
            n102 = register-events(w310, w306, w305) -> (reference out=w311:refnum<event-registration>, error out=w303:errorcluster)  [unwired: 2 in]
            n103 = Merge Errors(w303, w302, w301, w300, w299) -> (w309:errorcluster)
            n104 = call <vilib>:"Add State(s) to Queue__jki_lib_state_machine.vi"("State(s) in (\"\")"=w314) -> ("States Out"=w313:string)  [unwired: 14 in]
          }
          frame "Events: Unregister" {
            n105 = Unregister For Events(event registration refnum=w317, error in=w316) -> (error out=w315:errorcluster)
            n106 = call <vilib>:"Add State(s) to Queue__jki_lib_state_machine.vi"("State(s) in (\"\")"=w320) -> ("States Out"=w319:string)  [unwired: 14 in]
          }
          frame "---------- Action ----------" {
            n107 = Unbundle By Name(w323) -> ("Core.Last Error"=w321:T9)
            n108 = Bundle By Name(cluster=w323, "Core.Last Error"=w321) -> (w322:T4)
            n109 = call <vilib>:"Add State(s) to Queue__jki_lib_state_machine.vi"("State(s) in (\"\")"=w327) -> ("States Out"=w326:string)  [unwired: 14 in]
          }
          frame "Action: Notify UI Closed" {
            # "Notify that the UI has been closed"
            n110 = Unbundle By Name(w330) -> ("SelfRef"=w331:refnum<class "Instrument UI.Cryostation.lvclass">)
            n111 = call <vilib>:"Hide.vi"("error in (no error)"=w329, "SMO.UI"=w331) -> ("error out"=w328:errorcluster)  [unwired: 8 in, 1 out]
            n112 = call <vilib>:"Add State(s) to Queue__jki_lib_state_machine.vi"("State(s) in (\"\")"=w334) -> ("States Out"=w333:string)  [unwired: 14 in]
          }
        }
      }
    }
    frame Error {
    }
  }
  n113 = call-parent "Process.vi"("error in"=w5, "Instrument UI in"=w4) -> ("error out"=w2:errorcluster, "Instrument UI out"=→"Instrument.Cryostation UI":refnum<class "Instrument UI.Cryostation.lvclass">)  [unwired: 8 in]
  n114 = Merge Errors(w2, w1) -> (→"error out":errorcluster)
